vi "Automatic-Approach-Retraction-MCL-2013-04-28-1a-data-storage-1b1.vi"() -> ()   [LabVIEW 2012]
uses:
  <vilib>/rvi/Emulation/niFpgaSctlEmulationGetInTimedLoop.vi
  <vilib>/rvi/Emulation/niFpgaSctlEmulationGlobalWrite.vi
  <vilib>/rvi/interface/RandomDataEmulation/nirviRandomDataFPGAFIFO.vi
  <vilib>/rvi/interface/RandomDataEmulation/niFpgaRandomDataHandleErrors.vi
  <vilib>/rvi/eio/common/nirviEmuTemplateMethod_errors.vi
  <vilib>/rvi/DataTransferAndStorage/Container/XNode/niFpgaContainer.xnode
  <vilib>/rvi/interface/RandomDataEmulation/nirviRandomDataFpgaReadWriteTemplate.vi
  <vilib>/eio/EIONode/EIONode.xnode
  <vilib>/rvi/Analysis/measure/butterworth/XNode/niFpgaButterworthFilter.xnode
panel:
  out "TF-drift":i16
  out "Tick Count(Ticks)":u32=3198398528
  in  "Data Acquisition Rate (usec)":u32=500000
  out "Data storage":bool=TRUE
  out "Start Approach indicator":bool
  out "safetip minimum indicator":bool
  out "Data counter":u16
  out "Counter Output":i16
  in  "Initial Position":i16
  in  "phase 1 control":bool
  in  "Manual Control":bool
  in  "Zposition MCL fine 2":i16
  in  "MCL counter 2":u16
  out "Curve indicator":u16
  in  "Number of curves":u16
  out "TF Freq shift":i16
  in  "Timeout FIFO":i32=-1
  out "Phase 2":bool
  in  "Parameter":i16
  out "Phase 1":bool
  in  "Start Approach":bool
  out "MCL counter in range?":bool
  in  "Wait-tip-before-new-approach (usec)":u32
  in  "Fast Retraction After Cycle":i32
  in  "Wait-tip-before-approach":u32
  in  "Fast Retraction before approach":i32
  in  "Offset for Fast Approach":i16
  in  "Fast Approach (usec)":u32
  in  "Minimum for Approach Value":i16
  out "digital steps per region":u16
  in  "MCL Divisions":u16
  in  "MCL counter":u16
  in  "Fine Retraction (usec)":u32
  in  "TF at infinity":i16
  out "TF Phase Signal":i16(graph)
  out "Control Signal":i16
  in  "Fine Approach (usec)":u32
  in  "Setpoint Fine":i16
  out "Zposition MCL fine":i16
  in  "Initial Height (Fine)":i16=9113
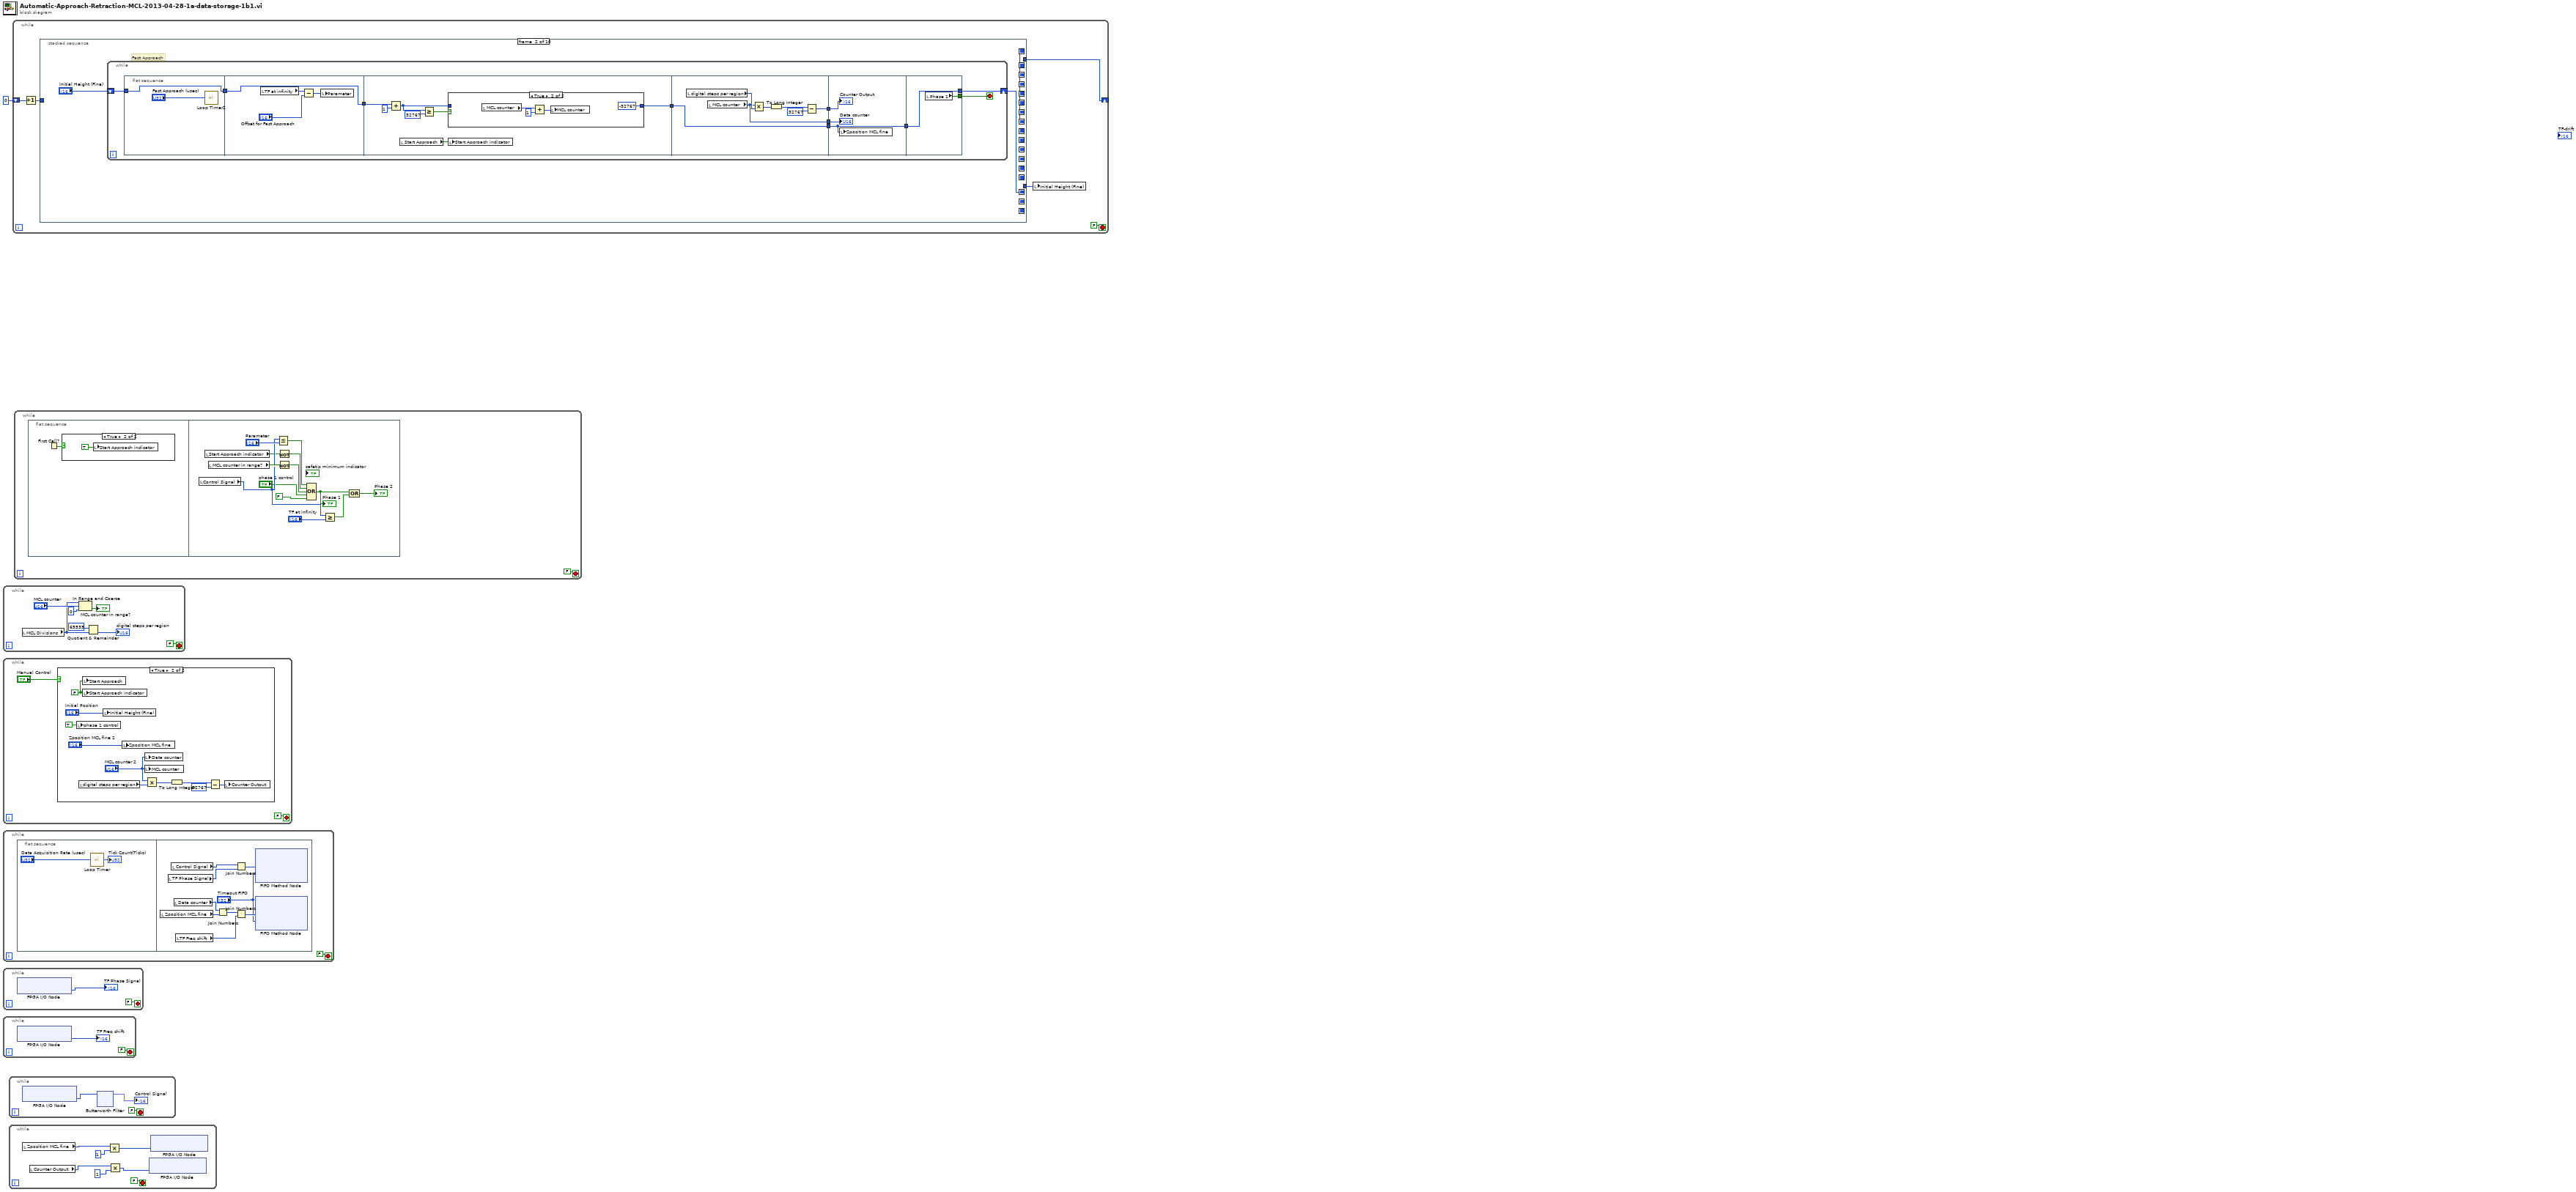
[diagram p0: block diagram]
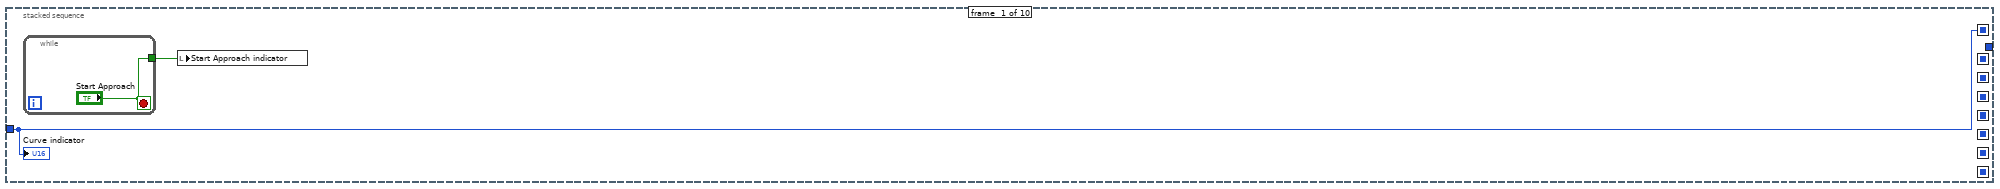
[diagram p4: hidden frame]
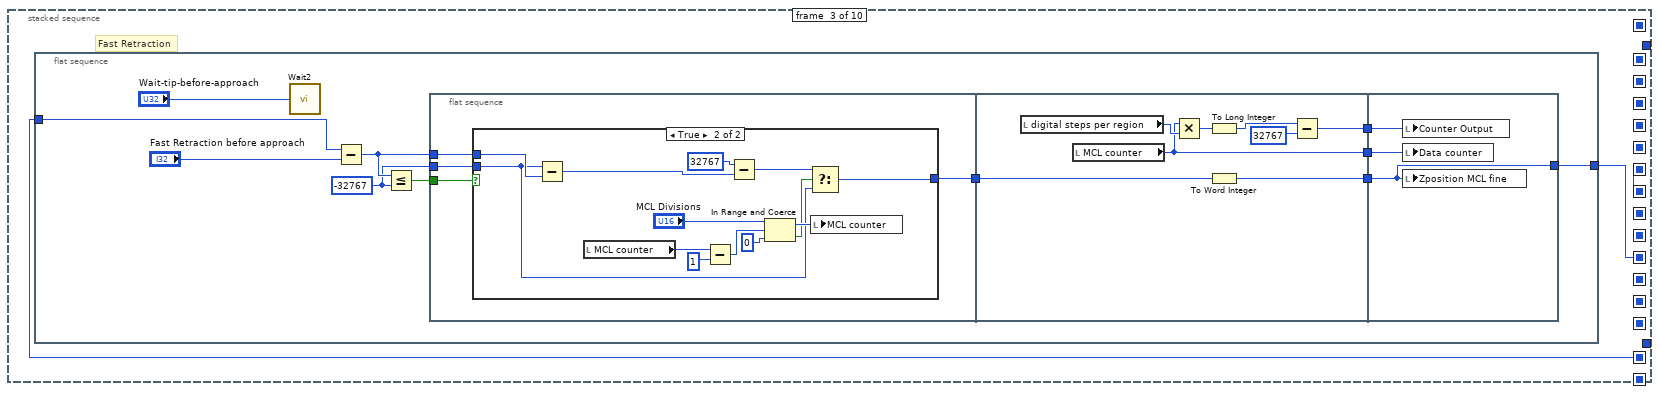
[diagram p6: hidden frame]
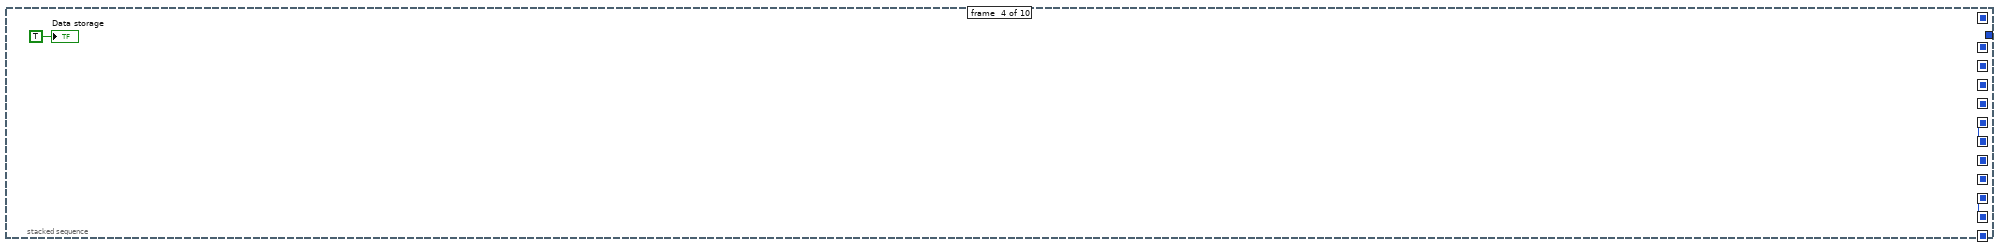
[diagram p8: hidden frame]
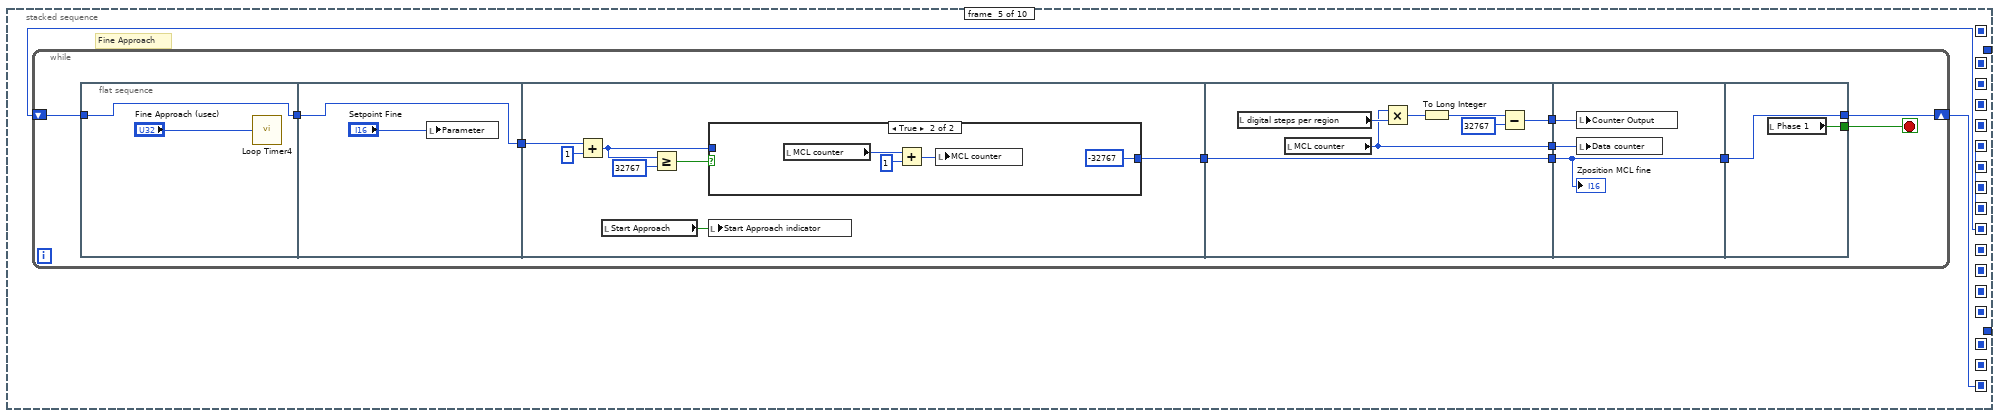
[diagram p9: hidden frame]
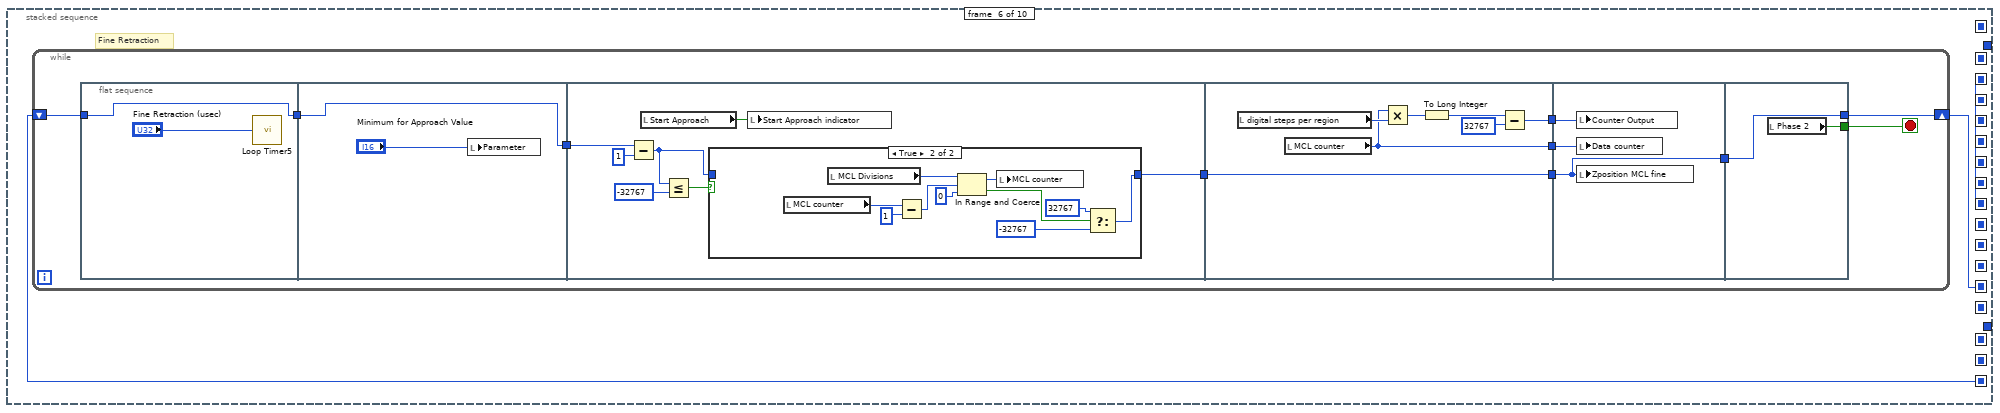
[diagram p11: hidden frame]
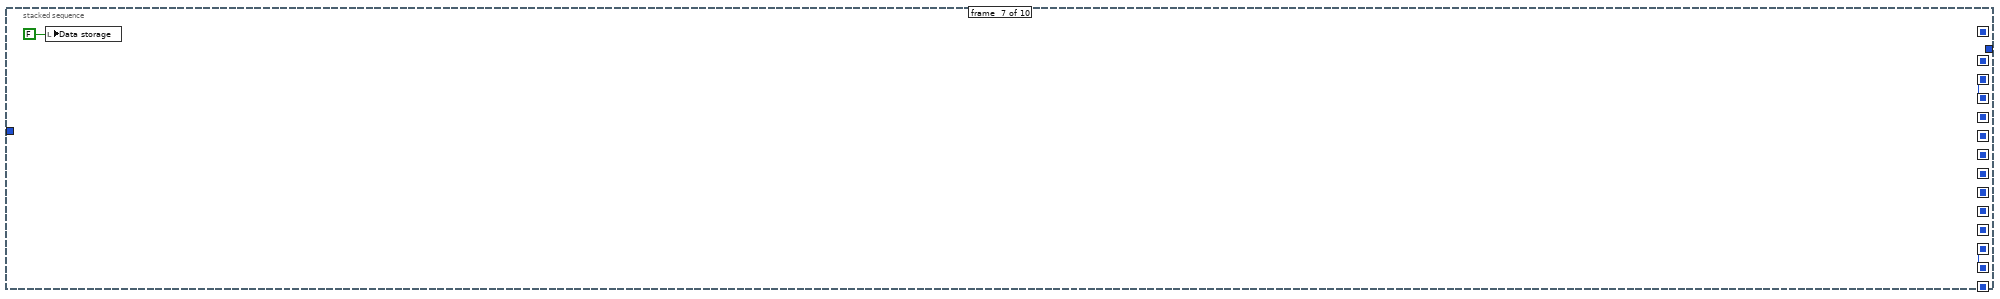
[diagram p13: hidden frame]
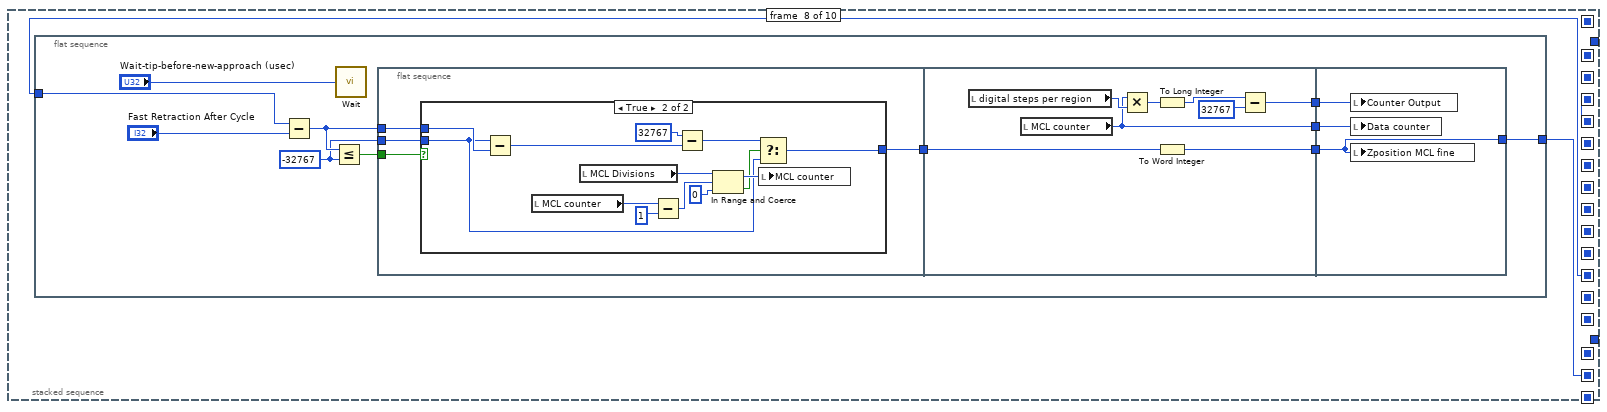
[diagram p14: hidden frame]
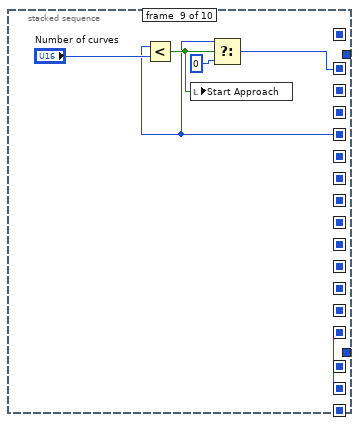
[diagram p16: hidden frame]
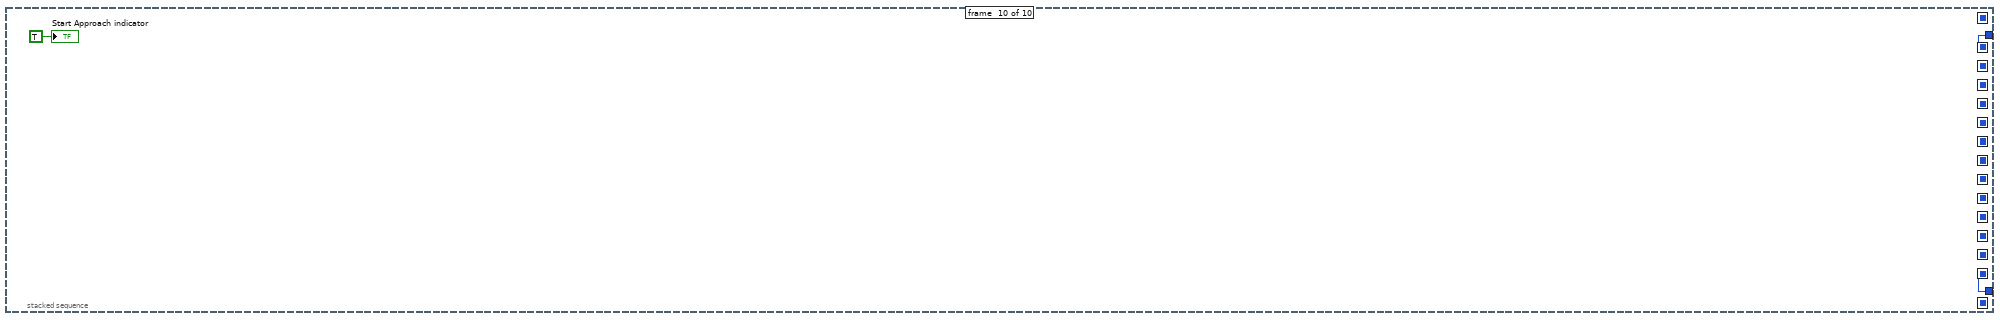
[diagram p17: hidden frame]
diagram:
  n1 = while {
    stop <- FALSE stop-if-true
    n2 = local read "MCL Divisions"() -> (w2:u16)
    n3 = In Range and Coerce(upper limit=w2, x="MCL counter", lower limit=u16 0) -> (In Range?=→"MCL counter in range?":bool)  [unwired: 1 out]
    n4 = Quotient & Remainder(x=65535, y=w2) -> (floor(x/y)=→"digital steps per region":i32)  [unwired: 1 out]
  }
  n5 = while {
    stop <- FALSE stop-if-true
    n6 = case shown="True" "Manual Control" {
      frame False {
      }
      frame True {
        w11 = FALSE ("Start Approach")
        n7 = local write "phase 1 control"(TRUE ("phase 1 control")) -> ()
        n8 = local read "digital steps per region"() -> (w17:u16)
        n9 = local write "Start Approach"(w11) -> ()
        n10 = local write "Start Approach indicator"(w11) -> ()
        n11 = local write "Initial Height (Fine)"("Initial Position") -> ()
        n12 = local write "Zposition MCL fine"("Zposition MCL fine 2") -> ()
        n13 = local write "Data counter"("MCL counter 2") -> ()
        n14 = local write "MCL counter"("MCL counter 2") -> ()
        n15 = Multiply(x="MCL counter 2", y=w17) -> (x*y=w13:u16)
        n16 = To Long Integer(number=w13) -> (32bit integer=w12:i32)
        n17 = Subtract(x=w12, y=32767) -> (x-y=w15:i32)
        n18 = local write "Counter Output"(w15) -> ()
      }
    }
  }
  n19 = while {
    stop <- FALSE stop-if-true
    n20 = flat-sequence {
      frame #0 {
        n21 = call "Loop Timer"("Count(Ticks)"="Data Acquisition Rate (usec)") -> ("Tick Count(Ticks)"=→"Tick Count(Ticks)":u32)
      }
      frame #1 {
        n22 = local read "Zposition MCL fine"() -> (w30:i16)
        n23 = local read "TF Phase Signal"() -> (w25:i16)
        n24 = local read "Control Signal"() -> (w26:i16)
        n25 = local read "Data counter"() -> (w31:u16)
        n26 = local read "TF Freq shift"() -> (w24:i16)
        n27 = Join Numbers(hi=w31, lo=w30) -> ((hi.lo)=w29:u32)
        n28 = Join Numbers(hi=w26, lo=w25) -> ((hi.lo)=w32:u32)
        n29 = Join Numbers(hi=w29, lo=w24) -> ((hi.lo)=w28:u64)
        n30 = xnode ("FIFO Method Node")("Element"=w32, "Timeout"="Timeout FIFO") -> ()  [unwired: 1 in, 2 out]
        n31 = xnode ("FIFO Method Node")("Element"=w28, "Timeout"="Timeout FIFO") -> ()  [unwired: 1 in, 2 out]
      }
    }
  }
  n32 = while {
    stop <- FALSE stop-if-true
    n33 = xnode "FPGA I/O Node"() -> ("Connector0/AI1"=→"TF Phase Signal":i16)  [unwired: 1 in, 1 out]
  }
  n34 = while {
    stop <- FALSE stop-if-true
    n35 = xnode "FPGA I/O Node"() -> ("Connector0/AI2"=→"TF Freq shift":i16)  [unwired: 1 in, 1 out]
  }
  n36 = while {
    stop <- FALSE stop-if-true
    n37 = xnode "FPGA I/O Node"() -> ("Connector0/AI7"=w38:i16)  [unwired: 1 in, 1 out]
    n38 = xnode "Butterworth Filter"("input data"=w38) -> ("output data"=→"Control Signal":fxp<+/-,20,20>)  [unwired: 2 in]
  }
  n39 = while {
    stop <- FALSE stop-if-true
    n40 = local read "Zposition MCL fine"() -> (w52:i16)
    n41 = local read "Counter Output"() -> (w48:i16)
    n42 = Multiply(x=w52, y=i16 1) -> (x*y=w51:i16)
    n43 = Multiply(x=w48, y=i16 1) -> (x*y=w49:i16)
    n44 = xnode "FPGA I/O Node"("Connector0/AO2"=w49) -> ()  [unwired: 1 in, 1 out]
    n45 = xnode "FPGA I/O Node"("Connector0/AO7"=w51) -> ()  [unwired: 1 in, 1 out]
  }
  n46 = while {
    shift-right: [w55] -> _
    shift-left: u16 0 ("t") -> [w54]
    stop <- FALSE stop-if-true
    n47 = Increment(x=w54) -> (x+1=w56:u16)
    n48 = stacked-sequence {
      seq-local: [w60 _ _ _ _ _ _ _ _ _] -> [_ w63 _ _ _ _ _ _ _ _]
      seq-local: [_ w64 _ _ _ _ _ _ _ _] -> [_ _ w107 _ _ _ _ _ _ _]
      seq-local: [_ w63 _ _ _ _ _ _ _ _] -> [_ _ w105 _ _ _ _ _ _ _]
      seq-local: [_ _ w106 _ _ _ _ _ _ _] -> [_ _ _ w150 _ _ _ _ _ _]
      seq-local: [_ _ w105 _ _ _ _ _ _ _] -> [_ _ _ w149 _ _ _ _ _ _]
      seq-local: [_ _ _ w150 _ _ _ _ _ _] -> [_ _ _ _ w153 _ _ _ _ _]
      seq-local: [_ _ _ w149 _ _ _ _ _ _] -> [_ _ _ _ w151 _ _ _ _ _]
      seq-local: [_ _ _ _ w152 _ _ _ _ _] -> [_ _ _ _ _ w194 _ _ _ _]
      seq-local: [_ _ _ _ w151 _ _ _ _ _] -> [_ _ _ _ _ w192 _ _ _ _]
      seq-local: [_ _ _ _ _ w193 _ _ _ _] -> [_ _ _ _ _ _ w241 _ _ _]
      seq-local: [_ _ _ _ _ w192 _ _ _ _] -> [_ _ _ _ _ _ w240 _ _ _]
      seq-local: [_ _ _ _ _ _ w241 _ _ _] -> [_ _ _ _ _ _ _ w244 _ _]
      seq-local: [_ _ _ _ _ _ w240 _ _ _] -> [_ _ _ _ _ _ _ w242 _ _]
      seq-local: [_ _ _ _ _ _ _ w243 _ _] -> [_ _ _ _ _ _ _ _ w290 _]
      seq-local: [_ _ _ _ _ _ _ w242 _ _] -> [_ _ _ _ _ _ _ _ w285 _]
      seq-local: [_ _ _ _ _ _ _ _ w290 _] -> [_ _ _ _ _ _ _ _ _ w293]
      seq-local: [_ _ _ _ _ _ _ _ w286 _] -> [_ _ _ _ _ _ _ _ _ w292]
      tunnel: w56 -> [w60 _ _ _ _ _ _ _ _ _]
      tunnel: [_ _ _ _ _ _ _ _ _ w293] -> w58
      tunnel: [_ _ _ _ _ _ _ _ _ w292] -> w55
      frame #0 {
        n49 = while {
          tunnel: ["Start Approach"] -> w59
          stop <- "Start Approach" stop-if-true
        }
        n50 = local write "Start Approach indicator"(w59) -> ()
        "Curve indicator" <- w60
      }
      frame #1 {
        # "Fast Approach"
        n51 = while {
          shift-right: [w73] -> w64
          shift-left: "Initial Height (Fine)" -> [w74]
          stop <- w69 stop-if-true
          n52 = flat-sequence {
            tunnel: w74 -> [w76]
            tunnel: [w76] -> w71
            tunnel: [w80] -> w72
            tunnel: w71 -> [w80]
            tunnel: [w86] -> w68
            tunnel: w72 -> [w87]
            tunnel: w68 -> [w99]
            tunnel: [w99] -> w67
            tunnel: [w96] -> w66
            tunnel: [w95] -> w65
            tunnel: w67 -> [w102]
            tunnel: [w102] -> w70
            tunnel: w66 -> [w101]
            tunnel: w65 -> [w100]
            tunnel: [w104] -> w73
            tunnel: w70 -> [w104]
            tunnel: [w103] -> w69
            frame #0 {
              n53 = call "Loop Timer2"("Count(uSec)"="Fast Approach (usec)") -> ()  [unwired: 1 out]
            }
            frame #1 {
              n54 = local read "TF at infinity"() -> (w77:i16)
              n55 = Subtract(x=w77, y="Offset for Fast Approach") -> (x-y=w79:i16)
              n56 = local write "Parameter"(w79) -> ()
            }
            frame #2 {
              n57 = Add(x=w87, y=i16 1) -> (x+y=w82:i16)
              n58 = local read "Start Approach"() -> (w81:bool)
              n59 = Greater Or Equal?(x=w82, y=i16 32767) -> (x >= y?=w83:bool)
              n60 = case shown="True" w83 {
                tunnel: [w88 i16 -32767] -> w86
                tunnel: w82 -> [w88 _]
                frame False {
                }
                frame True {
                  n61 = local read "MCL counter"() -> (w90:u16)
                  n62 = Add(x=w90, y=u16 1) -> (x+y=w89:u16)
                  n63 = local write "MCL counter"(w89) -> ()
                }
              }
              n64 = local write "Start Approach indicator"(w81) -> ()
            }
            frame #3 {
              n65 = local read "digital steps per region"() -> (w98:u16)
              n66 = local read "MCL counter"() -> (w95:u16)
              n67 = Multiply(x=w95, y=w98) -> (x*y=w94:u16)
              n68 = To Long Integer(number=w94) -> (32bit integer=w93:i32)
              n69 = Subtract(x=w93, y=32767) -> (x-y=w96:i32)
            }
            frame #4 {
              n70 = local write "Zposition MCL fine"(w102) -> ()
              "Counter Output" <- w101
              "Data counter" <- w100
            }
            frame #5 {
              n71 = local read "Phase 1"() -> (w103:bool)
            }
          }
        }
      }
      frame #2 {
        # "Fast Retraction"
        n72 = flat-sequence {
          tunnel: [w114] -> w106
          tunnel: w107 -> [w115]
          frame #0 {
            w112 = -32767 ("y")
            n73 = call "Wait2"("Count(uSec)"="Wait-tip-before-approach") -> ()  [unwired: 1 out]
            n74 = Subtract(x=w115, y="Fast Retraction before approach") -> (x-y=w117:i32)
            n75 = Less Or Equal?(x=w117, y=w112) -> (x <= y?=w118:bool)
            n76 = flat-sequence {
              tunnel: w118 -> [w122]
              tunnel: w117 -> [w121]
              tunnel: w112 -> [w119]
              tunnel: [w120] -> w111
              tunnel: w111 -> [w140]
              tunnel: [w139] -> w110
              tunnel: [w141] -> w109
              tunnel: [w142] -> w108
              tunnel: [w147] -> w114
              tunnel: w110 -> [w147]
              tunnel: w109 -> [w146]
              tunnel: w108 -> [w145]
              frame #0 {
                n77 = case shown="True" w122 {
                  tunnel: w121 -> [w123 w133]
                  tunnel: [w123 w125] -> w120
                  tunnel: w119 -> [_ w124]
                  frame False {
                  }
                  frame True {
                    n78 = Subtract(x=w124, y=w133) -> (x-y=w132:i32)
                    n79 = local read "MCL counter"() -> (w136:u16)
                    n80 = Subtract(x=w136, y=u16 1) -> (x-y=w129:u16)
                    n81 = Subtract(x=32767, y=w132) -> (x-y=w126:i32)
                    n82 = In Range and Coerce(upper limit="MCL Divisions", x=w129, lower limit=u16 0 ("upper limit")) -> (coerced(x)=w128:u16, In Range?=w127:bool)
                    n83 = Select(t=w126, s=w127, f=w124) -> (s? t:f=w125:i32)
                    n84 = local write "MCL counter"(w128) -> ()
                  }
                }
              }
              frame #1 {
                n85 = local read "digital steps per region"() -> (w144:u16)
                n86 = local read "MCL counter"() -> (w141:u16)
                n87 = Multiply(x=w141, y=w144) -> (x*y=w138:u16)
                n88 = To Long Integer(number=w138) -> (32bit integer=w137:i32)
                n89 = To Word Integer(number=w140) -> (16bit integer=w139:i16)
                n90 = Subtract(x=w137, y=32767) -> (x-y=w142:i32)
              }
              frame #2 {
                n91 = local write "Counter Output"(w145) -> ()
                n92 = local write "Data counter"(w146) -> ()
                n93 = local write "Zposition MCL fine"(w147) -> ()
              }
            }
          }
        }
      }
      frame #3 {
        "Data storage" <- TRUE
      }
      frame #4 {
        # "Fine Approach"
        n94 = while {
          shift-right: [w162] -> w152
          shift-left: w153 -> [w163]
          stop <- w154 stop-if-true
          n95 = flat-sequence {
            tunnel: w163 -> [w165]
            tunnel: [w165] -> w160
            tunnel: [w167] -> w161
            tunnel: w160 -> [w167]
            tunnel: [w173] -> w159
            tunnel: w161 -> [w174]
            tunnel: w159 -> [w186]
            tunnel: [w186] -> w158
            tunnel: [w183] -> w157
            tunnel: [w182] -> w156
            tunnel: w158 -> [w187]
            tunnel: w157 -> [w189]
            tunnel: w156 -> [w188]
            tunnel: [w187] -> w155
            tunnel: [w191] -> w162
            tunnel: w155 -> [w191]
            tunnel: [w190] -> w154
            frame #0 {
              n96 = call "Loop Timer4"("Count(uSec)"="Fine Approach (usec)") -> ()  [unwired: 1 out]
            }
            frame #1 {
              n97 = local write "Parameter"("Setpoint Fine") -> ()
            }
            frame #2 {
              n98 = Add(x=w174, y=i16 1) -> (x+y=w169:i16)
              n99 = local read "Start Approach"() -> (w168:bool)
              n100 = Greater Or Equal?(x=w169, y=i16 32767) -> (x >= y?=w170:bool)
              n101 = case shown="True" w170 {
                tunnel: [w175 i16 -32767] -> w173
                tunnel: w169 -> [w175 _]
                frame False {
                }
                frame True {
                  n102 = local read "MCL counter"() -> (w176:u16)
                  n103 = Add(x=w176, y=u16 1) -> (x+y=w178:u16)
                  n104 = local write "MCL counter"(w178) -> ()
                }
              }
              n105 = local write "Start Approach indicator"(w168) -> ()
            }
            frame #3 {
              n106 = local read "digital steps per region"() -> (w185:u16)
              n107 = local read "MCL counter"() -> (w182:u16)
              n108 = Multiply(x=w182, y=w185) -> (x*y=w181:u16)
              n109 = To Long Integer(number=w181) -> (32bit integer=w180:i32)
              n110 = Subtract(x=w180, y=32767) -> (x-y=w183:i32)
            }
            frame #4 {
              n111 = local write "Counter Output"(w189) -> ()
              n112 = local write "Data counter"(w188) -> ()
              "Zposition MCL fine" <- w187
            }
            frame #5 {
              n113 = local read "Phase 1"() -> (w190:bool)
            }
          }
        }
      }
      frame #5 {
        # "Fine Retraction"
        n114 = while {
          shift-right: [w203] -> w193
          shift-left: w194 -> [w204]
          stop <- w197 stop-if-true
          n115 = flat-sequence {
            tunnel: w204 -> [w206]
            tunnel: [w206] -> w200
            tunnel: [w208] -> w201
            tunnel: w200 -> [w208]
            tunnel: [w214] -> w202
            tunnel: w201 -> [w215]
            tunnel: w202 -> [w233]
            tunnel: [w233] -> w199
            tunnel: [w228] -> w196
            tunnel: [w227] -> w195
            tunnel: w199 -> [w234]
            tunnel: [w234] -> w198
            tunnel: w196 -> [w236]
            tunnel: w195 -> [w235]
            tunnel: [w238] -> w203
            tunnel: w198 -> [w238]
            tunnel: [w237] -> w197
            frame #0 {
              n116 = call "Loop Timer5"("Count(uSec)"="Fine Retraction (usec)") -> ()  [unwired: 1 out]
            }
            frame #1 {
              n117 = local write "Parameter"("Minimum for Approach Value") -> ()
            }
            frame #2 {
              n118 = Subtract(x=w215, y=i16 1) -> (x-y=w210:i16)
              n119 = local read "Start Approach"() -> (w209:bool)
              n120 = Less Or Equal?(x=w210, y=i16 -32767) -> (x <= y?=w212:bool)
              n121 = case shown="True" w212 {
                tunnel: w210 -> [w216 _]
                tunnel: [w216 w217] -> w214
                frame False {
                }
                frame True {
                  n122 = local read "MCL counter"() -> (w226:u16)
                  n123 = local read "MCL Divisions"() -> (w224:u16)
                  n124 = Subtract(x=w226, y=u16 1) -> (x-y=w222:u16)
                  n125 = In Range and Coerce(upper limit=w224, x=w222, lower limit=u16 0) -> (coerced(x)=w221:u16, In Range?=w220:bool)
                  n126 = local write "MCL counter"(w221) -> ()
                  n127 = Select(t=i16 32767, s=w220, f=i16 -32767) -> (s? t:f=w217:i16)
                }
              }
              n128 = local write "Start Approach indicator"(w209) -> ()
            }
            frame #3 {
              n129 = local read "digital steps per region"() -> (w232:u16)
              n130 = local read "MCL counter"() -> (w228:u16)
              n131 = Multiply(x=w228, y=w232) -> (x*y=w230:u16)
              n132 = To Long Integer(number=w230) -> (32bit integer=w229:i32)
              n133 = Subtract(x=w229, y=32767) -> (x-y=w227:i32)
            }
            frame #4 {
              n134 = local write "Counter Output"(w235) -> ()
              n135 = local write "Data counter"(w236) -> ()
              n136 = local write "Zposition MCL fine"(w234) -> ()
            }
            frame #5 {
              n137 = local read "Phase 2"() -> (w237:bool)
            }
          }
        }
      }
      frame #6 {
        n138 = local write "Data storage"(FALSE ("Data storage")) -> ()
      }
      frame #7 {
        n139 = flat-sequence {
          tunnel: [w251] -> w243
          tunnel: w244 -> [w252]
          frame #0 {
            w249 = -32767 ("y")
            n140 = Subtract(x=w252, y="Fast Retraction After Cycle") -> (x-y=w255:i32)
            n141 = Less Or Equal?(x=w255, y=w249) -> (x <= y?=w254:bool)
            n142 = call "Wait"("Count(uSec)"="Wait-tip-before-new-approach (usec)") -> ()  [unwired: 1 out]
            n143 = flat-sequence {
              tunnel: w255 -> [w259]
              tunnel: w254 -> [w258]
              tunnel: w249 -> [w256]
              tunnel: [w257] -> w248
              tunnel: w248 -> [w277]
              tunnel: [w276] -> w247
              tunnel: [w279] -> w246
              tunnel: [w278] -> w245
              tunnel: [w283] -> w251
              tunnel: w247 -> [w283]
              tunnel: w246 -> [w284]
              tunnel: w245 -> [w282]
              frame #0 {
                n144 = case shown="True" w258 {
                  tunnel: w259 -> [w260 w271]
                  tunnel: [w260 w261] -> w257
                  tunnel: w256 -> [_ w262]
                  frame False {
                  }
                  frame True {
                    n145 = Subtract(x=w262, y=w271) -> (x-y=w270:i32)
                    n146 = local read "MCL counter"() -> (w273:u16)
                    n147 = local read "MCL Divisions"() -> (w267:u16)
                    n148 = Subtract(x=w273, y=u16 1) -> (x-y=w268:u16)
                    n149 = Subtract(x=32767, y=w270) -> (x-y=w263:i32)
                    n150 = In Range and Coerce(upper limit=w267, x=w268, lower limit=u16 0) -> (coerced(x)=w265:u16, In Range?=w264:bool)
                    n151 = Select(t=w263, s=w264, f=w262) -> (s? t:f=w261:i32)
                    n152 = local write "MCL counter"(w265) -> ()
                  }
                }
              }
              frame #1 {
                n153 = local read "digital steps per region"() -> (w281:u16)
                n154 = local read "MCL counter"() -> (w278:u16)
                n155 = Multiply(x=w278, y=w281) -> (x*y=w275:u16)
                n156 = To Long Integer(number=w275) -> (32bit integer=w274:i32)
                n157 = To Word Integer(number=w277) -> (16bit integer=w276:i16)
                n158 = Subtract(x=w274, y=32767) -> (x-y=w279:i32)
              }
              frame #2 {
                n159 = local write "Counter Output"(w284) -> ()
                n160 = local write "Data counter"(w282) -> ()
                n161 = local write "Zposition MCL fine"(w283) -> ()
              }
            }
          }
        }
      }
      frame #8 {
        n162 = Less?(x=w285, y="Number of curves") -> (x < y?=w288:bool)
        n163 = local write "Start Approach"(w288) -> ()
        n164 = Select(t=w285, s=w288, f=u16 0 ("t")) -> (s? t:f=w286:u16)
      }
      frame #9 {
        "Start Approach indicator" <- TRUE ("Start Approach indicator")
      }
    }
    n165 = local write "Initial Height (Fine)"(w58) -> ()
  }
  n166 = while {
    stop <- FALSE stop-if-true
    n167 = flat-sequence {
      frame #0 {
        n168 = First Call?() -> (First Call?: T/F=w295:bool)
        n169 = case shown="True" w295 {
          frame False {
          }
          frame True {
            n170 = local write "Start Approach indicator"(TRUE ("Start Approach indicator")) -> ()
          }
        }
      }
      frame #1 {
        n171 = local read "Control Signal"() -> (w301:i16)
        n172 = local read "Start Approach indicator"() -> (w298:bool)
        n173 = local read "MCL counter in range?"() -> (w308:bool)
        n174 = Less Or Equal?(x=w301, y="Parameter") -> (x <= y?=w306:bool)
        n175 = Not(x=w298) -> (.not. x?=w307:bool)
        n176 = Not(x=w308) -> (.not. x?=w309:bool)
        n177 = Compound Arithmetic op=OR(w306, w307, w309, "phase 1 control", FALSE) -> (w299:bool)
        "Phase 1" <- w299
        n178 = Greater Or Equal?(x=w301, y="TF at infinity") -> (x >= y?=w303:bool)
        n179 = Compound Arithmetic op=OR(w299, w303) -> (→"Phase 2":bool)
      }
    }
  }
